vi "contrl.vi"() -> ()   [LabVIEW 2015]
uses:
  Ctrls/Main vari.ctl
  Ctrls/data out array.ctl
  Ctrls/data out.ctl
  Mode/config/CHS.ctl
  Mode/config/singlechtype.ctl
  Ctrls/command.ctl
  TCPIP/TCPIP_enum.ctl
  TCPIP/TCPIPconfig.ctl
panel:
  out "DRIVE_UNIT 2":string
  out "LOAD_UNIT 2":string
  in  "D":dbl
  in  "I":dbl
  in  "P":dbl
  out "LOAD_UNIT":string
  out "DRIVE_UNIT":string
  in  "D":dbl
  in  "I":dbl=0.1
  in  "P":dbl=2.0
  out "转速":dbl
  in  "sinmod":enum16{"Vmode", "Tmode", "ConPMote", "PNMote"}(ring)
  out "loader":cluster{dbl, dbl}(graph)
  out "driver":cluster{dbl, dbl}(graph)
  in  "load freq":dbl caption="load value"
  in  "driver freq":dbl caption="driver value"
  out "drive  V":dbl
  out "扭矩":dbl
  out "时间":timestamp format="%<%x %X>T"
  in  "loader Stop":bool
  in  "dirver Stop":bool
  out "Load Data":dbl format="%#_6f"
  in  "load_set":T1
  in  "load value":dbl format="%#.2g"
  in  "Settings_load":bool caption="Settings_driver"
  in  "Play_load":bool caption="Play_driver"
  in  "LOAD MODE":T2(ring) caption="模式选择"
  out "state_loader":T3 caption="state_load"
  out "Drive Data":dbl format="%#_6f"
  in  "driver_set":T1
  in  "driver value":dbl
  in  "Settings_driver":bool
  in  "Play_driver":bool
  in  "driver MODE":T4(ring) caption="模式选择"
  out "state_driver":T3
  in  "command":T5=22 items=["NO_Action", "start", "pause", "resum", "stop", "config", "System_constant", "7", "DAQ_init", "DAQ_config", "DAQ_start", "DAQ_read", "DAQ_stop", "DAQ_contrl", "14", "15", "16", "setting", "MODE_STOP", "P_MODE_RUN", "V_MODE_RUN", "T_MODE_RUN", "Sin_MODE_RUN", "Sin_MODE_STOP", "P_PN_RUN", "P_Con_RUN"]
  out "error out":errorcluster
  out "LED":bool[](array[boolean])
  in  "Query":bool
  in  "Exit":bool
  in  "Acquire":bool
  in  "Config":bool
  in  "Main Vari":T6={"Error"={"status"=FALSE, "code"=0, "source"=""}, "Test Info"={"Test Name"="", "Tester"=""}, "StateName"="", "Display Info"=[{"Frequency"=0.0, "RMS"=0.0}, {"Frequency"=0.0, "RMS"=0.0}, {"Frequency"=0.0, "RMS"=0.0}, {"Frequency"=0.0, "RMS"=0.0}, {"Frequency"=0.0, "RMS"=0.0}], "ch size"=0, "data out"=[], "CHS"=[], "CalData"=[]} {"CHS"."display" format="%b"}
  # "电机驱动控制系统"
  # "位置"
  # "速度"
  # "PID参数配置"
  # "力矩"
  # "速度"
  # "PID参数配置"
  # "Measurement System Ver 1.0  Copyright  by M_tech design studio"
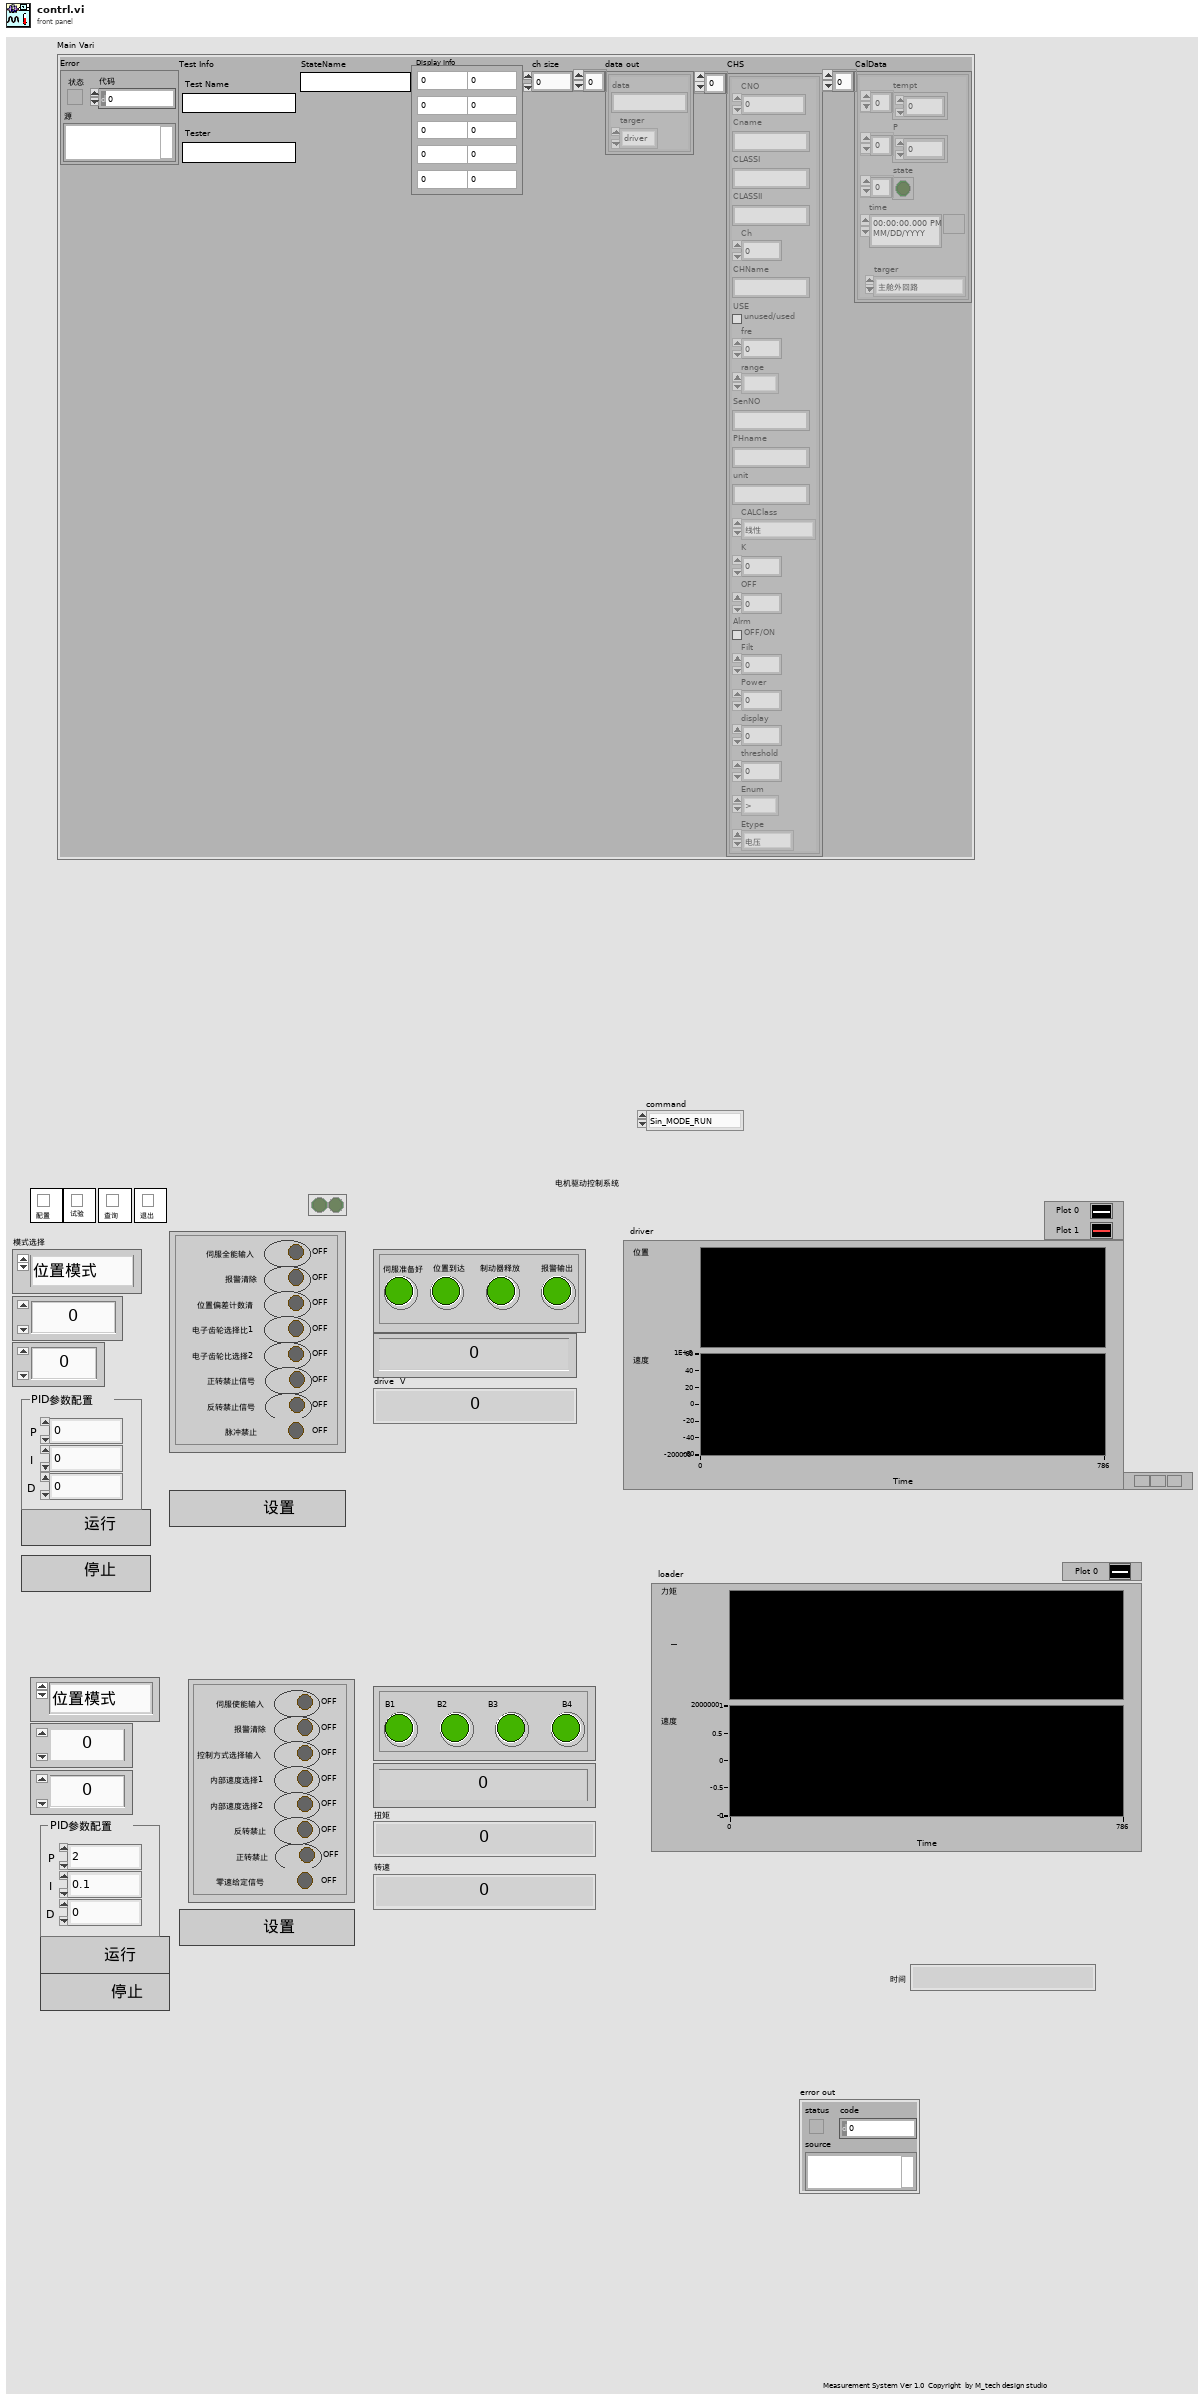
[diagram p1: front panel]
types:
  T1 = cluster{"set":bool, "set 2":bool, "set 3":bool, "set 4":bool, "set 5":bool, "set 6":bool, "set 7":bool, "set 8":bool}
  T2 = enum16{"位置模式", "速度模式", "力矩模式", "正弦力矩", "正弦速度", "PID恒力矩模式"}
  T3 = cluster{"B1":bool, "B2":bool, "B3":bool, "B4":bool}
  T4 = enum16{"位置模式", "速度模式", "力矩模式", "正弦力矩", "正弦速度", "正反转", "连续旋转"}
  T5 = typedef "command.ctl" = u16
  T6 = typedef "Main vari.ctl" = cluster{"Error":errorcluster, "Test Info":cluster{"Test Name":string, "Tester":string}, "StateName":string, "Display Info":T7, "ch size":u8, "data out":T8, "CHS":T10, "CalData":cluster{"tempt":dbl[], "P":dbl[], "state":bool[], "time":timestamp, "targer":enum16{"主舱外回路", "主舱内回路", "实验舱外回路", "实验舱内回路"}}[]}
  T7 = typedef "Display Information_Ctrls-某型振动实验台测试系统.ctl" = cluster{"Frequency":dbl, "RMS":dbl}[]
  T8 = typedef "data out array.ctl" = T9[]
  T9 = typedef "data out.ctl" = cluster{"data":string, "targer":enum16{"driver", "loader"}}
  T10 = typedef "CHS.ctl" = T11[]
  T11 = typedef "singlechtype.ctl" = cluster{"CNO":u8, "Cname":string, "CLASSI":string, "CLASSII":string, "Ch":u8, "CHName":string, "USE":bool, "fre":dbl, "range":enum16{""}, "SenNO":string, "PHname":string, "unit":string, "CALClass":enum8{"线性", "查表", "公式"}, "K":dbl, "OFF":dbl, "Alrm":bool, "Filt":dbl, "Power":u8, "display":u8, "threshold ":dbl, "Enum":enum16{">", ">=", "<", "<=", "<>(在范围内）", "><（在范围外）"}, "Etype":enum16{"电压", "电流", "电阻", "热电偶K", "热电偶T"}}
  T12 = typedef "Enum queue_Ctrls-某型振动实验台测试系统.ctl" = enum16{"Noop", "Send Pro1", "Send data", "Get Pro1", "Get data", "Flush Pro1", "Flush data", "Destroy Pro1", "Destroy data"}
  T13 = typedef "TCPIP_enum.ctl" = enum16{"init", "connect", "command", "write", "read", "close", "null"}
  T14 = cluster{"value":dbl, "freq":dbl, "sinmod":enum16{"Vmode", "Tmode"}}
  T15 = cluster{"value":dbl, "freq":dbl, "sinmod":enum16{"Vmode", "Tmode", "ConPMote", "PNMote"}, "P":dbl, "I":dbl, "D":dbl}
  T16 = cluster{"value":dbl, "freq":dbl, "sinmod":enum16{"Vmode", "Tmode", "PIDTmode"}, "P":dbl, "I":dbl, "D":dbl}
  T17 = typedef "TCPIPconfig.ctl" = cluster{"add":string, "port":u32, "timeout":u16, "connection ID":refnum<k5>, "targer":enum16{"driver", "loader"}}[]
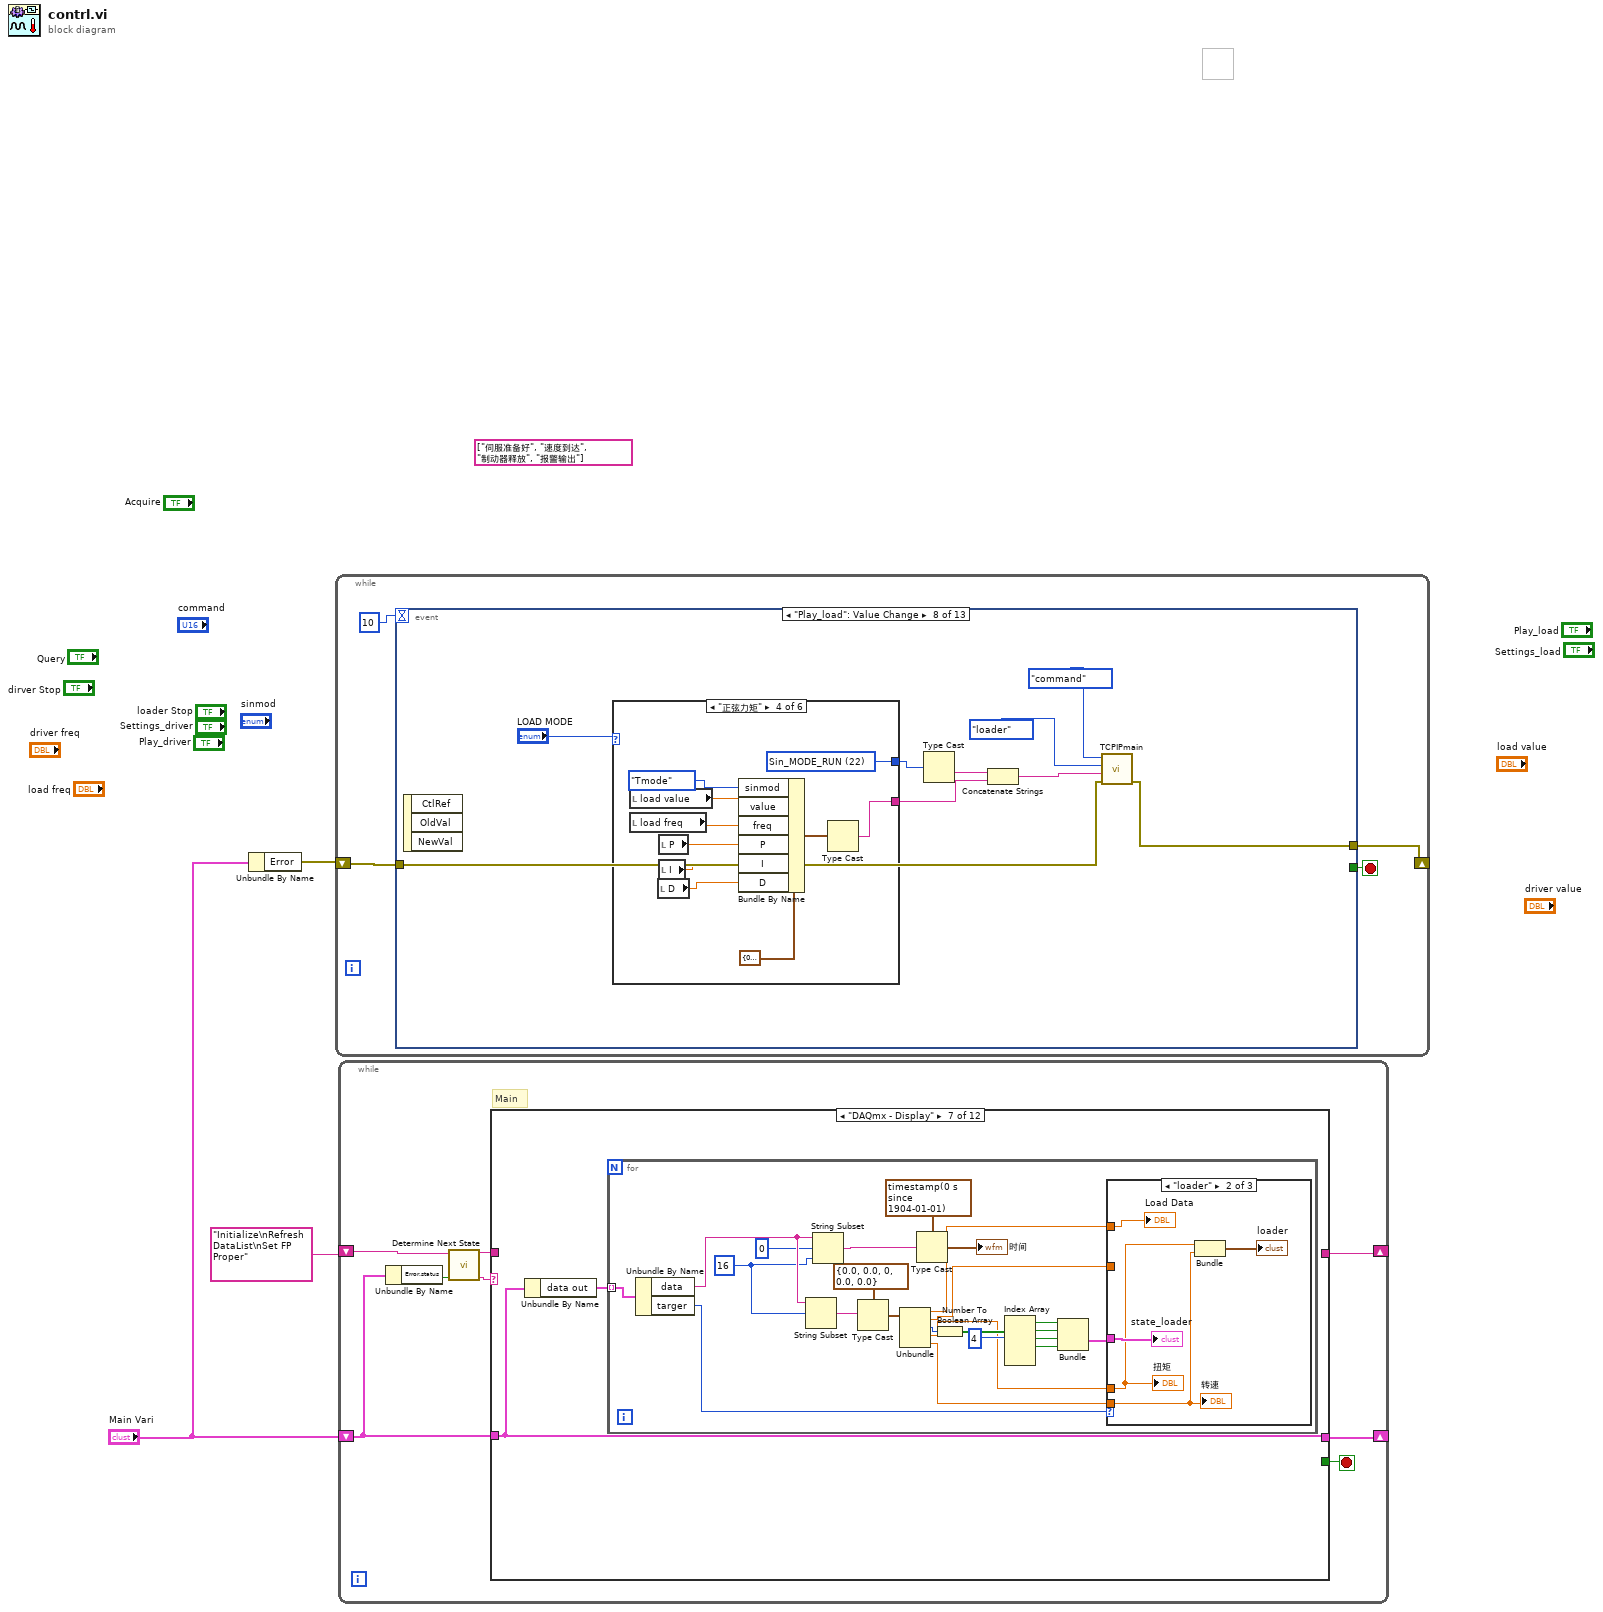
[diagram p0: block diagram]
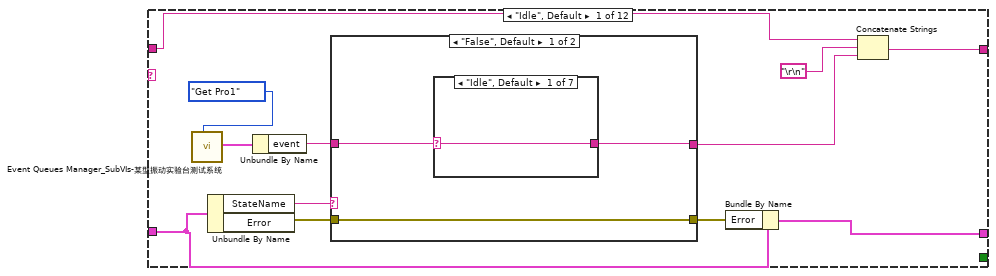
[diagram p2: hidden frame]
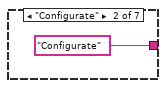
[diagram p3: hidden frame]
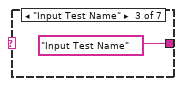
[diagram p4: hidden frame]
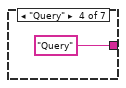
[diagram p5: hidden frame]
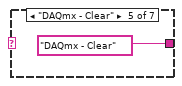
[diagram p6: hidden frame]
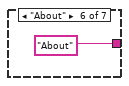
[diagram p7: hidden frame]
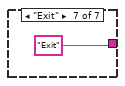
[diagram p8: hidden frame]
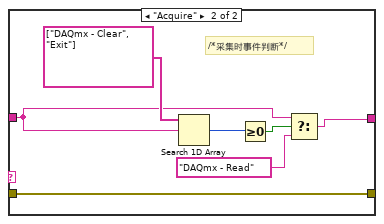
[diagram p9: hidden frame]
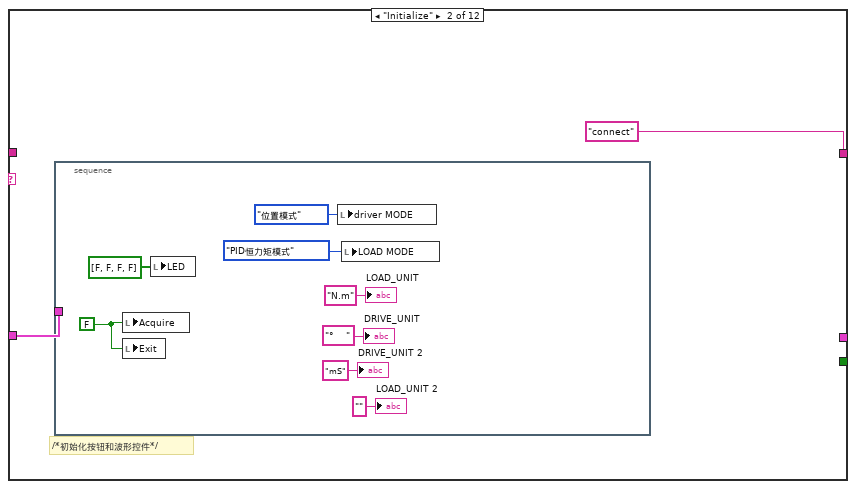
[diagram p10: hidden frame]
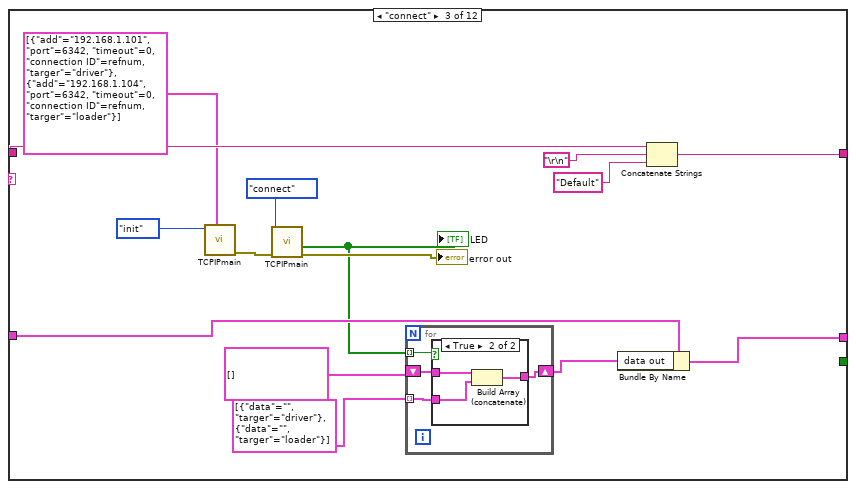
[diagram p11: hidden frame]
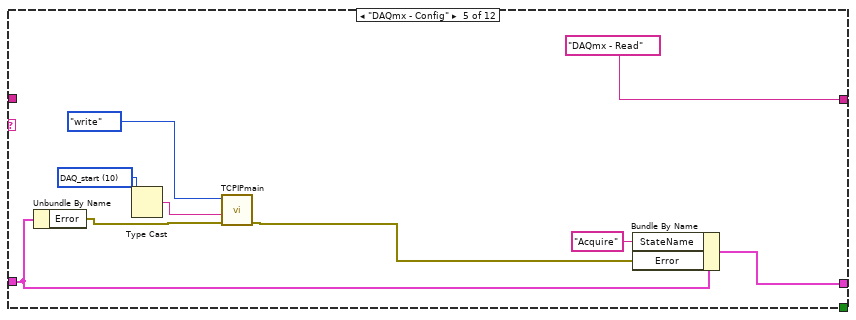
[diagram p14: hidden frame]
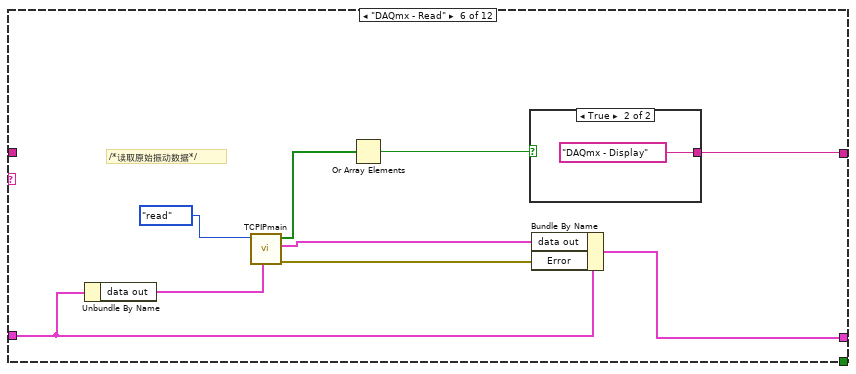
[diagram p15: hidden frame]
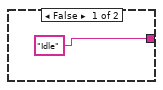
[diagram p16: hidden frame]
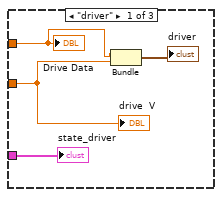
[diagram p17: hidden frame]
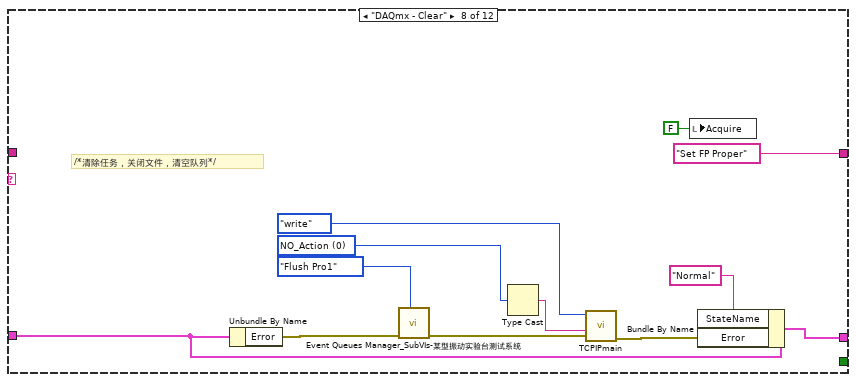
[diagram p19: hidden frame]
diagram:
  (unwired) string[] ["伺服准备好", "速度到达", "制动器释放", "报警输出"]
  n1 = Unbundle By Name("Main Vari") -> ("Error"=w1:errorcluster)
  n2 = while {
    shift-right: [w6] -> _
    shift-left: w1 -> [w7]
    stop <- w4 stop-if-true
    n3 = event shown="[7] \"Play_load\": Value Change" {
      selector: _ -> [_ _ _ _ _ _ _ _ _ _ _ _ _]
      dyn-events: _ -> [_ _ _ _ _ _ _ _ _ _ _ _ _]
      timeout: 10 -> [_ _ _ _ _ _ _ _ _ _ _ _ _]
      tunnel: w7 -> [w8 w14 w19 w30 w41 _ _ w167 w221 w232 w238 w244 w248]
      tunnel: [w9 w13 w18 w29 w40 _ _ w166 w210 w233 w239 w245 w247] -> w6
      tunnel: [_ _ w17 _ _ _ _ _ _ _ _ _ TRUE] -> w4
      event Timeout {
        # "/*判断是否有错误发生，若有错误发生，\n进入错误处理状态*/"
        n4 = event-data() -> ()  [unwired: 3 out]
        n5 = case shown="No Error" w8 {
          selector: w8 -> [w10 w11]
          tunnel: [w10 w12] -> w9
          frame No Error {
          }
          frame Error {
            n6 = call "Error Handle_SubVIs-某型振动实验台测试系统.vi"("error in"=w11) -> ("error out"=w12:errorcluster)  [unwired: 10 out]
          }
        }
      }
      event "Config": Value Change {
        # "/*若配置键被按下，进入到配置状态中*/"
        n7 = event-data() -> ()  [unwired: 2 out]
        n8 = call "Event Queues Manager_SubVIs-某型振动实验台测试系统.vi"("Mode"=Enum_queue_Ctrls-某型振动实验台测试系统."Send Pro1" ("Mod"), "error in"=w14, "event"="Configurate") -> ("error out"=w13:errorcluster)  [unwired: 2 in, 6 out]
      }
      event Menu Selection (User) {
        # "/*按照选中的菜单标签跳转到相应状态*/"
        n9 = event-data() -> ("ItemTag"=w20:string)  [unwired: 1 out]
        n10 = case shown="\"File - Configure\"" w20 {
          tunnel: [_ "Configurate" ("event") "Exit" ("event") "Input Test Name" ("event") "Query" ("event") "About" ("event")] -> w22
          tunnel: [_ _ TRUE _ _ _] -> w17
          frame "", Default {
          }
          frame "File - Configure" {
          }
          frame "Exit" {
          }
          frame "Operate - Run" {
          }
          frame "Operate - Query" {
          }
          frame "Help - About" {
          }
        }
        n11 = call "Event Queues Manager_SubVIs-某型振动实验台测试系统.vi"("Mode"=Enum_queue_Ctrls-某型振动实验台测试系统."Send Pro1" ("Mod"), "error in"=w19, "event"=w22) -> ("error out"=w18:errorcluster)  [unwired: 2 in, 6 out]
      }
      event "Acquire": Value Change {
        n12 = event-data() -> ("NewVal"=w35:bool)  [unwired: 1 out]
        n13 = Select(t="DAQmx - Config" ("event"), s=w35, f="DAQmx - Clear" ("event")) -> (s? t:f=w31:string)
        n14 = call "Event Queues Manager_SubVIs-某型振动实验台测试系统.vi"("Mode"=Enum_queue_Ctrls-某型振动实验台测试系统."Send Pro1" ("Mod"), "error in"=w30, "event"=w31) -> ("error out"=w29:errorcluster)  [unwired: 2 in, 6 out]
      }
      event "Play_driver": Value Change {
        n15 = event-data() -> ()  [unwired: 4 out]
        n16 = case shown="\"连续旋转\"" "driver MODE" {
          tunnel: [w47 w54 w61 w64 w67 w74 w84] -> w38
          tunnel: [w45 w53 w60 w62 w65 w73 w83] -> w37
          frame "位置模式", Default {
            w47 = T5 19 items=["NO_Action", "start", "pause", "resum", "stop", "config", "System_constant", "7", "DAQ_init", "DAQ_config", "DAQ_start", "DAQ_read", "DAQ_stop", "DAQ_contrl", "14", "15", "16", "setting", "MODE_STOP", "P_MODE_RUN", "V_MODE_RUN", "T_MODE_RUN"] ("command 2")
            n17 = local read "driver value"() -> (w46:dbl)
            n18 = Type Cast(x=w46) -> (*(type *) &x=w45:string)  [unwired: 1 in]
          }
          frame "正弦力矩" {
            w54 = T5 22 items=["NO_Action", "start", "pause", "resum", "stop", "config", "System_constant", "7", "DAQ_init", "DAQ_config", "DAQ_start", "DAQ_read", "DAQ_stop", "DAQ_contrl", "14", "15", "16", "setting", "MODE_STOP", "P_MODE_RUN", "V_MODE_RUN", "T_MODE_RUN", "Sin_MODE_RUN", "Sin_MODE_STOP"] ("command")
            n19 = local read "driver value"() -> (w51:dbl)
            n20 = local read "driver freq"() -> (w50:dbl)
            n21 = Bundle By Name(cluster=T14 {"value"=0.0, "freq"=0.0, "sinmod"=enum."Vmode"}, "sinmod"=enum16{"Vmode", "Tmode"}."Vmode", "value"=w51, "freq"=w50) -> (w52:T14)
            n22 = Type Cast(x=w52) -> (*(type *) &x=w53:string)  [unwired: 1 in]
          }
          frame "正弦速度" {
            w61 = T5 22 items=["NO_Action", "start", "pause", "resum", "stop", "config", "System_constant", "7", "DAQ_init", "DAQ_config", "DAQ_start", "DAQ_read", "DAQ_stop", "DAQ_contrl", "14", "15", "16", "setting", "MODE_STOP", "P_MODE_RUN", "V_MODE_RUN", "T_MODE_RUN", "Sin_MODE_RUN", "Sin_MODE_STOP"] ("command")
            n23 = local read "driver value"() -> (w58:dbl)
            n24 = local read "driver freq"() -> (w57:dbl)
            n25 = Bundle By Name(cluster=T14 {"value"=0.0, "freq"=0.0, "sinmod"=enum."Vmode"}, "sinmod"=enum16{"Vmode", "Tmode"}."Vmode", "value"=w58, "freq"=w57) -> (w59:T14)
            n26 = Type Cast(x=w59) -> (*(type *) &x=w60:string)  [unwired: 1 in]
          }
          frame "速度模式" {
            w64 = T5 20 items=["NO_Action", "start", "pause", "resum", "stop", "config", "System_constant", "7", "DAQ_init", "DAQ_config", "DAQ_start", "DAQ_read", "DAQ_stop", "DAQ_contrl", "14", "15", "16", "setting", "MODE_STOP", "P_MODE_RUN", "V_MODE_RUN", "T_MODE_RUN"] ("command 2")
            n27 = local read "driver value"() -> (w63:dbl)
            n28 = Type Cast(x=w63) -> (*(type *) &x=w62:string)  [unwired: 1 in]
          }
          frame "力矩模式" {
            w67 = T5 21 items=["NO_Action", "start", "pause", "resum", "stop", "config", "System_constant", "7", "DAQ_init", "DAQ_config", "DAQ_start", "DAQ_read", "DAQ_stop", "DAQ_contrl", "14", "15", "16", "setting", "MODE_STOP", "P_MODE_RUN", "V_MODE_RUN", "T_MODE_RUN"] ("command 2")
            n29 = local read "driver value"() -> (w66:dbl)
            n30 = Type Cast(x=w66) -> (*(type *) &x=w65:string)  [unwired: 1 in]
          }
          frame "连续旋转" {
            w74 = T5 22 items=["NO_Action", "start", "pause", "resum", "stop", "config", "System_constant", "7", "DAQ_init", "DAQ_config", "DAQ_start", "DAQ_read", "DAQ_stop", "DAQ_contrl", "14", "15", "16", "setting", "MODE_STOP", "P_MODE_RUN", "V_MODE_RUN", "T_MODE_RUN", "Sin_MODE_RUN", "Sin_MODE_STOP"] ("command")
            n31 = local read "driver value"() -> (w76:dbl)
            n32 = local read "driver freq"() -> (w75:dbl)
            n33 = local read "D"() -> (w68:dbl)
            n34 = local read "I"() -> (w69:dbl)
            n35 = local read "P"() -> (w70:dbl)
            n36 = Bundle By Name(cluster=T15 {"value"=0.0, "freq"=0.0, "sinmod"=enum."ConPMote", "P"=0.0, "I"=0.0, "D"=0.0}, "sinmod"=enum16{"Vmode", "Tmode", "ConPMote", "PNMote"}."ConPMote", "value"=w76, "freq"=w75, "P"=w70, "I"=w69, "D"=w68) -> (w77:T15)
            n37 = Type Cast(x=w77) -> (*(type *) &x=w73:string)  [unwired: 1 in]
          }
          frame "正反转" {
            w84 = T5 22 items=["NO_Action", "start", "pause", "resum", "stop", "config", "System_constant", "7", "DAQ_init", "DAQ_config", "DAQ_start", "DAQ_read", "DAQ_stop", "DAQ_contrl", "14", "15", "16", "setting", "MODE_STOP", "P_MODE_RUN", "V_MODE_RUN", "T_MODE_RUN", "Sin_MODE_RUN", "Sin_MODE_STOP"] ("command")
            n38 = local read "driver value"() -> (w86:dbl)
            n39 = local read "driver freq"() -> (w85:dbl)
            n40 = Bundle By Name(cluster=T15 {"value"=0.0, "freq"=0.0, "sinmod"=enum."ConPMote", "P"=0.0, "I"=0.0, "D"=0.0}, "sinmod"=enum16{"Vmode", "Tmode", "ConPMote", "PNMote"}."PNMote", "value"=w86, "freq"=w85, "P"="P", "I"="I", "D"="D") -> (w87:T15)
            n41 = Type Cast(x=w87) -> (*(type *) &x=w83:string)  [unwired: 1 in]
          }
        }
        n42 = Type Cast(x=w38) -> (*(type *) &x=w44:string)  [unwired: 1 in]
        n43 = Concatenate Strings(w44, w37) -> (w42:string)
        n44 = call "TCPIPmain.vi"("error in"=w41, "data in"=w42, "targer"=enum16{"driver", "loader"}."driver", "Enum"=TCPIP_enum."command") -> ("error out"=w40:errorcluster)  [unwired: 3 in, 3 out]
      }
      event "driver MODE": Value Change {
        n45 = event-data() -> ("NewVal"=w94:T4)  [unwired: 3 out]
        n46 = case shown="\"连续旋转\"" w94 {
          tunnel: [string[] ["伺服全能输入", "报警清除", "位置偏差计数清", "电子齿轮选择比1", "电子齿轮比选择2", "正转禁止信号", "反转禁止信号", "脉冲禁止"] string[] ["伺服使能输入", "报警清除", "内部速度选择1", "内部速度选择2", "内部速度选择3", "正转禁止", "反转禁止", "零速给定信号"] string[] ["伺服使能输入", "报警清除", "控制方式选择输入", "内部速度选择1", "内部速度选择2", "正转禁止", "反转禁止", "零速给定信号"] string[] ["伺服使能输入", "报警清除", "控制方式选择输入", "内部速度选择1", "内部速度选择2", "正转禁止", "反转禁止", "零速给定信号"] string[] ["伺服使能输入", "报警清除", "内部速度选择1", "内部速度选择2", "内部速度选择3", "正转禁止", "反转禁止", "零速给定信号"] string[] ["伺服全能输入", "报警清除", "位置偏差计数清", "电子齿轮选择比1", "电子齿轮比选择2", "正转禁止信号", "反转禁止信号", "脉冲禁止"] string[] ["伺服全能输入", "报警清除", "位置偏差计数清", "电子齿轮选择比1", "电子齿轮比选择2", "正转禁止信号", "反转禁止信号", "脉冲禁止"]] -> w92
          tunnel: [string[] ["伺服准备好", "位置到达", "制动器释放", "报警输出"] string[] ["伺服准备好", "速度到达", "制动器释放", "报警输出"] string[] ["B1", "B2", "B3", "B4"] string[] ["B1", "B2", "B3", "B4"] string[] ["伺服准备好", "速度到达", "制动器释放", "报警输出"] string[] ["伺服准备好", "位置到达", "制动器释放", "报警输出"] string[] ["伺服准备好", "位置到达", "制动器释放", "报警输出"]] -> w90
          tunnel: ["脉冲个数" "RPM" "N.m" "N.m" "RPM" "脉冲个数" "脉冲个数"] -> w89
          tunnel: ["" ("DRIVE_UNIT 2") "" ("DRIVE_UNIT 2") "" ("DRIVE_UNIT 2") "Hz" ("DRIVE_UNIT 2") "Hz" ("DRIVE_UNIT 2") "ms" ("DRIVE_UNIT 2") "mS   " ("DRIVE_UNIT 2")] -> w88
          frame "位置模式", Default {
            (unwired) string[] ["伺服全能输入", "报警清除", "位置偏差计数清", "电子齿轮选择比1", "电子齿轮比选择2", "正转禁止信号", "反转禁止信号", "脉冲禁止"]
          }
          frame "速度模式" {
          }
          frame "力矩模式" {
          }
          frame "正弦力矩" {
          }
          frame "正弦速度" {
          }
          frame "正反转" {
          }
          frame "连续旋转" {
          }
        }
        n47 = local write "DRIVE_UNIT 2"(w88) -> ()
        n48 = property on="driver_set" class="Clust (strict)"() -> ("Controls[]"=w93:refnum<vi>[])  [unwired: 2 in, 2 out]
        n49 = local write "DRIVE_UNIT"(w89) -> ()
        n50 = property on="state_driver" class="Clust (strict)"() -> ("Controls[]"=w91:refnum<vi>[])  [unwired: 2 in, 2 out]
        n51 = for {
          tunnel: w93 -> [w98] mode=indexing
          tunnel: w92 -> [w97] mode=indexing
          n52 = property class="Ctl"(reference=w98, "Caption.Text"=w97) -> ()  [unwired: 1 in, 2 out]
        }
        n53 = for {
          tunnel: w91 -> [w96] mode=indexing
          tunnel: w90 -> [w95] mode=indexing
          n54 = property class="Ctl"(reference=w96, "Caption.Text"=w95) -> ()  [unwired: 1 in, 2 out]
        }
      }
      event "LOAD MODE": Value Change {
        n55 = event-data() -> ("NewVal"=w131:T2)  [unwired: 3 out]
        n56 = case shown="\"正弦力矩\"" w131 {
          tunnel: [string[] ["伺服全能输入", "报警清除", "位置偏差计数清", "电子齿轮选择比1", "电子齿轮比选择2", "正转禁止信号", "反转禁止信号", "脉冲禁止"] string[] ["伺服使能输入", "报警清除", "内部速度选择1", "内部速度选择2", "内部速度选择3", "正转禁止", "反转禁止", "零速给定信号"] string[] ["伺服使能输入", "报警清除", "控制方式选择输入", "内部速度选择1", "内部速度选择2", "正转禁止", "反转禁止", "零速给定信号"] string[] ["伺服使能输入", "报警清除", "控制方式选择输入", "内部速度选择1", "内部速度选择2", "正转禁止", "反转禁止", "零速给定信号"] string[] ["伺服使能输入", "报警清除", "内部速度选择1", "内部速度选择2", "内部速度选择3", "正转禁止", "反转禁止", "零速给定信号"] string[] ["伺服使能输入", "报警清除", "控制方式选择输入", "内部速度选择1", "内部速度选择2", "正转禁止", "反转禁止", "零速给定信号"]] -> w132
          tunnel: [string[] ["伺服准备好", "位置到达", "制动器释放", "报警输出"] string[] ["伺服准备好", "速度到达", "制动器释放", "报警输出"] string[] ["B1", "B2", "B3", "B4"] string[] ["B1", "B2", "B3", "B4"] string[] ["伺服准备好", "速度到达", "制动器释放", "报警输出"] string[] ["B1", "B2", "B3", "B4"]] -> w129
          tunnel: ["脉冲个数" "RPM" "N.m" "N.m" "RPM" "N.m"] -> w128
          tunnel: ["" "" "" "Hz" "Hz" "mS"] -> w127
          frame "位置模式", Default {
          }
          frame "速度模式" {
          }
          frame "力矩模式" {
          }
          frame "正弦力矩" {
          }
          frame "正弦速度" {
          }
          frame "PID恒力矩模式" {
          }
        }
        n57 = local write "LOAD_UNIT"(w128) -> ()
        n58 = local write "LOAD_UNIT 2"(w127) -> ()
        n59 = property on="load_set" class="Clust (strict)"() -> ("Controls[]"=w133:refnum<vi>[])  [unwired: 2 in, 2 out]
        n60 = property on="state_loader" class="Clust (strict)"() -> ("Controls[]"=w130:refnum<vi>[])  [unwired: 2 in, 2 out]
        n61 = for {
          tunnel: w133 -> [w161] mode=indexing
          tunnel: w132 -> [w160] mode=indexing
          n62 = property class="Ctl"(reference=w161, "Caption.Text"=w160) -> ()  [unwired: 1 in, 2 out]
        }
        n63 = for {
          tunnel: w130 -> [w135] mode=indexing
          tunnel: w129 -> [w134] mode=indexing
          n64 = property class="Ctl"(reference=w135, "Caption.Text"=w134) -> ()  [unwired: 1 in, 2 out]
        }
      }
      event "Play_load": Value Change {
        n65 = event-data() -> ()  [unwired: 4 out]
        n66 = case shown="\"正弦力矩\"" "LOAD MODE" {
          tunnel: [w173 w176 w179 w189 w199 w209] -> w164
          tunnel: [w171 w174 w177 w188 w198 w208] -> w162
          frame "位置模式", Default {
            w173 = T5 19 items=["NO_Action", "start", "pause", "resum", "stop", "config", "System_constant", "7", "DAQ_init", "DAQ_config", "DAQ_start", "DAQ_read", "DAQ_stop", "DAQ_contrl", "14", "15", "16", "setting", "MODE_STOP", "P_MODE_RUN", "V_MODE_RUN", "T_MODE_RUN"] ("command 2")
            n67 = local read "load value"() -> (w172:dbl)
            n68 = Type Cast(x=w172) -> (*(type *) &x=w171:string)  [unwired: 1 in]
          }
          frame "速度模式" {
            w176 = T5 20 items=["NO_Action", "start", "pause", "resum", "stop", "config", "System_constant", "7", "DAQ_init", "DAQ_config", "DAQ_start", "DAQ_read", "DAQ_stop", "DAQ_contrl", "14", "15", "16", "setting", "MODE_STOP", "P_MODE_RUN", "V_MODE_RUN", "T_MODE_RUN"] ("command 2")
            n69 = local read "load value"() -> (w175:dbl)
            n70 = Type Cast(x=w175) -> (*(type *) &x=w174:string)  [unwired: 1 in]
          }
          frame "力矩模式" {
            w179 = T5 21 items=["NO_Action", "start", "pause", "resum", "stop", "config", "System_constant", "7", "DAQ_init", "DAQ_config", "DAQ_start", "DAQ_read", "DAQ_stop", "DAQ_contrl", "14", "15", "16", "setting", "MODE_STOP", "P_MODE_RUN", "V_MODE_RUN", "T_MODE_RUN"] ("command 2")
            n71 = local read "load value"() -> (w178:dbl)
            n72 = Type Cast(x=w178) -> (*(type *) &x=w177:string)  [unwired: 1 in]
          }
          frame "正弦力矩" {
            w189 = T5 22 items=["NO_Action", "start", "pause", "resum", "stop", "config", "System_constant", "7", "DAQ_init", "DAQ_config", "DAQ_start", "DAQ_read", "DAQ_stop", "DAQ_contrl", "14", "15", "16", "setting", "MODE_STOP", "P_MODE_RUN", "V_MODE_RUN", "T_MODE_RUN", "Sin_MODE_RUN", "Sin_MODE_STOP"] ("command")
            n73 = local read "load value"() -> (w187:dbl)
            n74 = local read "load freq"() -> (w186:dbl)
            n75 = local read "D"() -> (w180:dbl)
            n76 = local read "P"() -> (w182:dbl)
            n77 = local read "I"() -> (w181:dbl)
            n78 = Bundle By Name(cluster=T16 {"value"=0.0, "freq"=0.0, "sinmod"=enum."PIDTmode", "P"=0.0, "I"=0.0, "D"=0.0}, "sinmod"=enum16{"Vmode", "Tmode", "PIDTmode"}."Tmode", "value"=w187, "freq"=w186, "P"=w182, "I"=w181, "D"=w180) -> (w185:T16)
            n79 = Type Cast(x=w185) -> (*(type *) &x=w188:string)  [unwired: 1 in]
          }
          frame "PID恒力矩模式" {
            w199 = T5 22 items=["NO_Action", "start", "pause", "resum", "stop", "config", "System_constant", "7", "DAQ_init", "DAQ_config", "DAQ_start", "DAQ_read", "DAQ_stop", "DAQ_contrl", "14", "15", "16", "setting", "MODE_STOP", "P_MODE_RUN", "V_MODE_RUN", "T_MODE_RUN", "Sin_MODE_RUN", "Sin_MODE_STOP"] ("command")
            n80 = local read "load value"() -> (w197:dbl)
            n81 = local read "load freq"() -> (w196:dbl)
            n82 = Bundle By Name(cluster=T16 {"value"=0.0, "freq"=0.0, "sinmod"=enum."PIDTmode", "P"=0.0, "I"=0.0, "D"=0.0}, "sinmod"=enum16{"Vmode", "Tmode", "PIDTmode"}."PIDTmode", "value"=w197, "freq"=w196, "P"="P", "I"="D", "D"="I") -> (w195:T16)
            n83 = Type Cast(x=w195) -> (*(type *) &x=w198:string)  [unwired: 1 in]
          }
          frame "正弦速度" {
            w209 = T5 22 items=["NO_Action", "start", "pause", "resum", "stop", "config", "System_constant", "7", "DAQ_init", "DAQ_config", "DAQ_start", "DAQ_read", "DAQ_stop", "DAQ_contrl", "14", "15", "16", "setting", "MODE_STOP", "P_MODE_RUN", "V_MODE_RUN", "T_MODE_RUN", "Sin_MODE_RUN", "Sin_MODE_STOP"] ("command")
            n84 = local read "load value"() -> (w207:dbl)
            n85 = local read "load freq"() -> (w206:dbl)
            n86 = local read "D"() -> (w200:dbl)
            n87 = local read "P"() -> (w202:dbl)
            n88 = local read "I"() -> (w201:dbl)
            n89 = Bundle By Name(cluster=T16 {"value"=0.0, "freq"=0.0, "sinmod"=enum."PIDTmode", "P"=0.0, "I"=0.0, "D"=0.0}, "sinmod"=enum16{"Vmode", "Tmode", "PIDTmode"}."Vmode", "value"=w207, "freq"=w206, "P"=w202, "I"=w201, "D"=w200) -> (w205:T16)
            n90 = Type Cast(x=w205) -> (*(type *) &x=w208:string)  [unwired: 1 in]
          }
        }
        n91 = Type Cast(x=w164) -> (*(type *) &x=w170:string)  [unwired: 1 in]
        n92 = Concatenate Strings(w170, w162) -> (w168:string)
        n93 = call "TCPIPmain.vi"("error in"=w167, "data in"=w168, "targer"=enum16{"driver", "loader"}."loader", "Enum"=TCPIP_enum."command") -> ("error out"=w166:errorcluster)  [unwired: 3 in, 3 out]
      }
      event "Settings_driver": Value Change {
        w214 = T5 17 items=["NO_Action", "start", "pause", "resum", "stop", "config", "System_constant", "7", "DAQ_init", "DAQ_config", "DAQ_start", "DAQ_read", "DAQ_stop", "DAQ_contrl", "14", "15", "16", "setting", "MODE_STOP", "P_MODE_RUN", "V_MODE_RUN", "T_MODE_RUN"] ("command")
        n94 = event-data() -> ()  [unwired: 2 out]
        n95 = Cluster To Array(cluster="driver_set") -> (array=w212:bool[])
        n96 = Boolean Array To Number(Boolean array=w212) -> (number=w211:u32)
        n97 = To Unsigned Byte Integer(number=w211) -> (unsigned 8bit integer=w216:u8)
        n98 = Type Cast(x=w214) -> (*(type *) &x=w218:string)  [unwired: 1 in]
        n99 = Type Cast(x=w216) -> (*(type *) &x=w217:string)  [unwired: 1 in]
        n100 = Concatenate Strings(w218, w217) -> (w220:string)
        n101 = call "TCPIPmain.vi"("error in"=w221, "data in"=w220, "targer"=enum16{"driver", "loader"}."driver", "Enum"=TCPIP_enum."command") -> ("error out"=w210:errorcluster)  [unwired: 3 in, 3 out]
      }
      event "Settings_load": Value Change {
        w225 = T5 17 items=["NO_Action", "start", "pause", "resum", "stop", "config", "System_constant", "7", "DAQ_init", "DAQ_config", "DAQ_start", "DAQ_read", "DAQ_stop", "DAQ_contrl", "14", "15", "16", "setting", "MODE_STOP", "P_MODE_RUN", "V_MODE_RUN", "T_MODE_RUN"] ("command")
        n102 = event-data() -> ()  [unwired: 2 out]
        n103 = Cluster To Array(cluster="load_set") -> (array=w223:bool[])
        n104 = Boolean Array To Number(Boolean array=w223) -> (number=w222:u32)
        n105 = To Unsigned Byte Integer(number=w222) -> (unsigned 8bit integer=w227:u8)
        n106 = Type Cast(x=w225) -> (*(type *) &x=w229:string)  [unwired: 1 in]
        n107 = Type Cast(x=w227) -> (*(type *) &x=w228:string)  [unwired: 1 in]
        n108 = Concatenate Strings(w229, w228) -> (w231:string)
        n109 = call "TCPIPmain.vi"("error in"=w232, "data in"=w231, "targer"=enum16{"driver", "loader"}."loader", "Enum"=TCPIP_enum."command") -> ("error out"=w233:errorcluster)  [unwired: 3 in, 3 out]
      }
      event "dirver Stop": Value Change {
        w234 = T5 23 items=["NO_Action", "start", "pause", "resum", "stop", "config", "System_constant", "7", "DAQ_init", "DAQ_config", "DAQ_start", "DAQ_read", "DAQ_stop", "DAQ_contrl", "14", "15", "16", "setting", "MODE_STOP", "P_MODE_RUN", "V_MODE_RUN", "T_MODE_RUN", "Sin_MODE_RUN", "Sin_MODE_STOP"] ("command")
        n110 = event-data() -> ()  [unwired: 2 out]
        n111 = Type Cast(x=w234) -> (*(type *) &x=w235:string)  [unwired: 1 in]
        n112 = call "TCPIPmain.vi"("error in"=w238, "data in"=w235, "targer"=enum16{"driver", "loader"}."driver", "Enum"=TCPIP_enum."command") -> ("error out"=w239:errorcluster)  [unwired: 3 in, 3 out]
      }
      event "loader Stop": Value Change {
        w240 = T5 23 items=["NO_Action", "start", "pause", "resum", "stop", "config", "System_constant", "7", "DAQ_init", "DAQ_config", "DAQ_start", "DAQ_read", "DAQ_stop", "DAQ_contrl", "14", "15", "16", "setting", "MODE_STOP", "P_MODE_RUN", "V_MODE_RUN", "T_MODE_RUN", "Sin_MODE_RUN", "Sin_MODE_STOP"] ("command")
        n113 = event-data() -> ()  [unwired: 2 out]
        n114 = Type Cast(x=w240) -> (*(type *) &x=w241:string)  [unwired: 1 in]
        n115 = call "TCPIPmain.vi"("error in"=w244, "data in"=w241, "targer"=enum16{"driver", "loader"}."loader", "Enum"=TCPIP_enum."command") -> ("error out"=w245:errorcluster)  [unwired: 3 in, 3 out]
      }
      event "Exit": Value Change {
        n116 = event-data() -> ()  [unwired: 2 out]
        n117 = call "Event Queues Manager_SubVIs-某型振动实验台测试系统.vi"("Mode"=Enum_queue_Ctrls-某型振动实验台测试系统."Send Pro1" ("Mod"), "error in"=w248, "event"="Exit") -> ("error out"=w247:errorcluster)  [unwired: 2 in, 6 out]
      }
    }
  }
  n118 = while {
    shift-right: [w257] -> _
    shift-left: "Main Vari" -> [w253]
    shift-right: [w255] -> _
    shift-left: "Initialize\nRefresh DataList\nSet FP Proper" ("Previous State") -> [w256]
    stop <- w258 stop-if-true
    # "Main"
    n119 = Unbundle By Name(w253) -> ("Error.status"=w252:bool)
    n120 = call "Determine Next State.vi"("Status?"=w252, "Previous State"=w256) -> ("New State"=w251:string, "Remaining States"=w254:string)  [unwired: 4 out]
    n121 = case shown="\"DAQmx - Display\"" w251 {
      tunnel: [_ _ _ _ _ _ _ _ _ _ _ TRUE] -> w258
      tunnel: w253 -> [w265 w289 w303 w322 w329 w334 w344 w383 w389 w395 w400 w403]
      tunnel: [w264 _ w304 w322 w330 w337 w344 w387 w389 w394 w399 w402] -> w257
      tunnel: [w261 "connect" ("Remaining States") w308 w321 "DAQmx - Read" ("event") w340 _ "Set FP Proper" ("Remaining States") w390 w391 w398 w401] -> w255
      tunnel: w254 -> [w262 _ w307 w321 _ _ _ _ w390 w391 w398 w401]
      frame "Idle", Default {
        n122 = call "Event Queues Manager_SubVIs-某型振动实验台测试系统.vi"("Mode"=Enum_queue_Ctrls-某型振动实验台测试系统."Get Pro1" ("Mod")) -> ("Process1"=w270:cluster{"event":string, "Message":variant})  [unwired: 4 in, 6 out]
        n123 = Unbundle By Name(w265) -> ("StateName"=w267:string, "Error"=w266:errorcluster)
        n124 = Unbundle By Name(w270) -> ("event"=w268:string)
        n125 = case shown="\"False\", Default" w267 {
          tunnel: w268 -> [w273 w284]
          tunnel: [w272 w283] -> w260
          tunnel: w266 -> [w271 w282]
          tunnel: [w271 w282] -> w263
          frame "False", Default {
            n126 = case shown="\"Idle\", Default" w273 {
              selector: w273 -> [w274 _ _ _ _ _ _]
              tunnel: [w274 "Configurate" ("Previous State") "Input Test Name" ("event") "Query" ("event") "DAQmx - Clear" ("event") "About" ("event") "Exit" ("event")] -> w272
              frame "Idle", Default {
              }
              frame "Configurate" {
              }
              frame "Input Test Name" {
              }
              frame "Query" {
              }
              frame "DAQmx - Clear" {
              }
              frame "About" {
              }
              frame "Exit" {
              }
            }
          }
          frame "Acquire" {
            # "/*采集时事件判断*/"
            n127 = Search 1D Array(1D array=string[] ["DAQmx - Clear", "Exit"], element=w284) -> (index of element=w286:i32)  [unwired: 1 out]
            n128 = Greater Or Equal To 0?(x=w286) -> (x >= 0?=w285:bool)
            n129 = Select(t=w284, s=w285, f="DAQmx - Read" ("event")) -> (s? t:f=w283:string)
          }
        }
        n130 = Bundle By Name(cluster=w265, "Error"=w263) -> (w264:T6)
        n131 = Concatenate Strings(w262, "\r\n", w260) -> (w261:string)
      }
      frame "Initialize" {
        # "/*初始化按钮和波形控件*/"
        n132 = stacked-sequence {
          tunnel: w289 -> [_]
          frame #0 {
            w297 = FALSE ("Start")
            n133 = local write "Acquire"(w297) -> ()
            n134 = local write "Exit"(w297) -> ()
            n135 = local write "LED"(bool[] [FALSE, FALSE, FALSE, FALSE] ("LED")) -> ()
            n136 = local write "driver MODE"(T4."位置模式" ("driver MODE")) -> ()
            n137 = local write "LOAD MODE"(T2."PID恒力矩模式" ("LOAD MODE")) -> ()
            "LOAD_UNIT" <- "N.m" ("LOAD_UNIT")
            "DRIVE_UNIT" <- "°    " ("LOAd_UNIT")
            "DRIVE_UNIT 2" <- "mS" ("DRIVE_UNIT 2")
            "LOAD_UNIT 2" <- "" ("LOAD_UNIT 2")
          }
        }
      }
      frame "connect" {
        n138 = call "TCPIPmain.vi"("config"=T17 [{"add"="192.168.1.101", "port"=6342, "timeout"=0, "connection ID"=refnum, "targer"=enum."driver"}, {"add"="192.168.1.104", "port"=6342, "timeout"=0, "connection ID"=refnum, "targer"=enum."loader"}], "Enum"=TCPIP_enum."init") -> ("error out"=w311:errorcluster)  [unwired: 5 in, 3 out]
        n139 = call "TCPIPmain.vi"("error in"=w311, "Enum"=TCPIP_enum."connect") -> ("error out"=→"error out":errorcluster, "LED"=w302:bool[])  [unwired: 5 in, 2 out]
        "LED" <- w302
        n140 = for {
          tunnel: w302 -> [w316] mode=indexing
          shift-right: [w313] -> w298
          shift-left: T9[] [] ("data out") -> [w315]
          tunnel: T9[] [{"data"="", "targer"=enum."driver"}, {"data"="", "targer"=enum."loader"}] ("data out") -> [w314] mode=indexing
          n141 = case shown="True" w316 {
            tunnel: w315 -> [w317 w320]
            tunnel: w314 -> [_ w319]
            tunnel: [w317 w318] -> w313
            frame False {
            }
            frame True {
              n142 = Build Array (concatenate)(w320, w319) -> (w318:T9[])
            }
          }
        }
        n143 = Bundle By Name(cluster=w303, "data out"=w298) -> (w304:T6)
        n144 = Concatenate Strings(w307, "\r\n", "Default" ("string")) -> (w308:string)
      }
      frame "-----------------" {
      }
      frame "DAQmx - Config" {
        w327 = T5 10 items=["NO_Action", "start", "pause", "resum", "stop", "config", "System_constant", "7", "DAQ_init", "DAQ_config", "DAQ_start", "DAQ_read", "DAQ_stop", "DAQ_contrl", "14", "15", "16", "17", "18", "19", ""] ("command")
        n145 = Unbundle By Name(w329) -> ("Error"=w328:errorcluster)
        n146 = Type Cast(x=w327) -> (*(type *) &x=w326:string)  [unwired: 1 in]
        n147 = call "TCPIPmain.vi"("error in"=w328, "data in"=w326, "Enum"=TCPIP_enum."write") -> ("error out"=w323:errorcluster)  [unwired: 4 in, 3 out]
        n148 = Bundle By Name(cluster=w329, "StateName"="Acquire", "Error"=w323) -> (w330:T6)
      }
      frame "DAQmx - Read" {
        # "/*读取原始振动数据*/"
        n149 = Unbundle By Name(w334) -> ("data out"=w332:T8)
        n150 = call "TCPIPmain.vi"("data"=w332, "Enum"=TCPIP_enum."read") -> ("error out"=w333:errorcluster, "data out"=w338:T8, "Data?"=w336:bool[])  [unwired: 5 in, 1 out]
        n151 = Or Array Elements(Boolean array=w336) -> (logical OR=w335:bool)
        n152 = case shown="True" w335 {
          tunnel: ["Idle" ("Remaining States") "DAQmx - Display" ("event")] -> w340
          frame False {
          }
          frame True {
          }
        }
        n153 = Bundle By Name(cluster=w334, "data out"=w338, "Error"=w333) -> (w337:T6)
      }
      frame "DAQmx - Display" {
        n154 = Unbundle By Name(w344) -> ("data out"=w343:T8)
        n155 = for {
          tunnel: w343 -> [w366] mode=indexing
          w364 = 16
          n156 = Unbundle By Name(w366) -> ("data"=w367:string, "targer"=w357:enum16{"driver", "loader"})
          n157 = String Subset(string=w367, offset (0)=w364) -> (substring=w361:string)  [unwired: 1 in]
          n158 = String Subset(string=w367, offset (0)=0, length (rest)=w364) -> (substring=w362:string)
          n159 = Type Cast(type=cluster{dbl, dbl, u8, dbl, dbl} {0.0, 0.0, 0, 0.0, 0.0}, x=w361) -> (*(type *) &x=w359:cluster{dbl, dbl, u8, dbl, dbl})
          n160 = Unbundle(w359) -> (w356:dbl, w346:dbl, w348:u8, w345:dbl, w347:dbl)
          n161 = Type Cast(type=timestamp(0 s since 1904-01-01), x=w362) -> (*(type *) &x=→"时间":timestamp)
          n162 = Number To Boolean Array(number=w348) -> (Boolean array=w358:bool[])
          n163 = Index Array(array=w358, index #1=4 ("index")) -> (element #1=w352:bool, element #2=w351:bool, element #3=w350:bool, element #4=w349:bool)  [unwired: 3 in]
          n164 = Bundle(w352, w351, w350, w349) -> (w355:cluster{bool, bool, bool, bool})  [unwired: 1 in]
          n165 = case shown="\"loader\"" w357 {
            tunnel: w356 -> [w370 w375 _]
            tunnel: w355 -> [w371 w376 _]
            tunnel: w345 -> [_ w373 _]
            tunnel: w347 -> [_ w372 _]
            tunnel: w346 -> [w368 _ _]
            frame "driver" {
              n166 = Bundle(w370, w368) -> (→"driver":cluster{dbl, dbl})  [unwired: 1 in]
              "Drive Data" <- w370
              "state_driver" <- w371
              "drive  V" <- w368
            }
            frame "loader" {
              n167 = Bundle(w373, w372) -> (→"loader":cluster{dbl, dbl})  [unwired: 1 in]
              "Load Data" <- w375
              "state_loader" <- w376
              "扭矩" <- w373
              "转速" <- w372
            }
            frame Default {
            }
          }
        }
      }
      frame "DAQmx - Clear" {
        w381 = T5 0 items=["NO_Action", "start", "pause", "resum", "stop", "config", "System_constant", "7", "DAQ_init", "DAQ_config", "DAQ_start", "DAQ_read", "DAQ_stop", "DAQ_contrl", "14", "15", "16", "17", "18", "19", ""] ("command")
        # "/*清除任务，关闭文件，清空队列*/"
        n168 = Unbundle By Name(w383) -> ("Error"=w377:errorcluster)
        n169 = call "Event Queues Manager_SubVIs-某型振动实验台测试系统.vi"("Mode"=Enum_queue_Ctrls-某型振动实验台测试系统."Flush Pro1" ("Mod"), "error in"=w377) -> ("error out"=w380:errorcluster)  [unwired: 3 in, 6 out]
        n170 = Type Cast(x=w381) -> (*(type *) &x=w382:string)  [unwired: 1 in]
        n171 = call "TCPIPmain.vi"("error in"=w380, "data in"=w382, "Enum"=TCPIP_enum."write") -> ("error out"=w378:errorcluster)  [unwired: 4 in, 3 out]
        n172 = local write "Acquire"(FALSE ("Acquire")) -> ()
        n173 = Bundle By Name(cluster=w383, "StateName"="Normal", "Error"=w378) -> (w387:T6)
      }
      frame "---------------------" {
      }
      frame "Error Handle" {
        # "/*若发生错误，进行错误处理*/"
        n174 = Unbundle By Name(w395) -> ("Error"=w393:errorcluster)
        n175 = call "Error Handle_SubVIs-某型振动实验台测试系统.vi"("error in"=w393) -> ("error out"=w392:errorcluster)  [unwired: 10 out]
        n176 = Bundle By Name(cluster=w395, "Error"=w392) -> (w394:T6)
      }
      frame "About" {
        n177 = Unbundle By Name(w400) -> ("Error"=w397:errorcluster)
        n178 = call "About.vi"("error in (no error)"=w397) -> ("error out"=w396:errorcluster)  [unwired: 10 out]
        n179 = Bundle By Name(cluster=w400, "Error"=w396) -> (w399:T6)
      }
      frame "Exit" {
        n180 = Unbundle By Name(w403) -> ("Error"=w405:errorcluster)
        n181 = call "Event Queues Manager_SubVIs-某型振动实验台测试系统.vi"("Mode"=Enum_queue_Ctrls-某型振动实验台测试系统."Destroy Pro1" ("Mod"), "error in"=w405) -> ("error out"=w404:errorcluster)  [unwired: 3 in, 6 out]
        n182 = Bundle By Name(cluster=w403, "Error"=w404) -> (w402:T6)
        n183 = disable-structure shown="Disabled" {
          frame Disabled {
            n184 = Quit LabVIEW(quit? (T)=TRUE) -> ()
          }
          frame Enabled {
          }
        }
      }
    }
  }
